vi "Read Current Limits.vi"   [LabVIEW 2023, in "Current Limits.lvclass"]
uses:
  Current Limits.lvclass
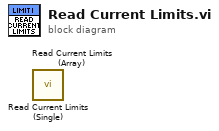
[diagram p0: block diagram]
diagram:
  n1 = call "Read Current Limits (Single).vi"() -> ()  [unwired: 7 in, 5 out]
  n2 = call "Read Current Limits (Array).vi"() -> ()  [unwired: 7 in, 5 out]
